vi "GET SV Variables from Target.vi"(7 "Read/Write":string, 8 "error in (no error)":errorcluster, 11 "Target":string) -> (0 "error out":errorcluster, 3 "Channel Array":refnum<class "ChannelVS.lvclass">[](array[class]))   [LabVIEW 2020, in "Shared Variables CD 2.0 Configuration.lvlib"]
uses:
  Shared Variables CD 2.0 Configuration.lvlib
  ChannelVS/ChannelVS.lvclass
  <vilib>/NI VeriStand/Custom Device API/Custom Device Item Ref.ctl
  ChannelVS/ChannelVS.lvclass/ChannelVS.ctl
  IPAddress Functions/ValidIPAddr.vi
  <vilib>/Utility/error.llb/Error Cluster From Error Code.vi
  Shared/SV Global.vi
  <resource>/objmgr/ni.var.rc
  built/windows/Channel.lvlibp/Channel.lvclass
  <vilib>/Utility/Data Type/NI_Data Type.lvlib
  <vilib>/NI VeriStand/Custom Device API/Custom Device API.lvlib
  C:/Users/Administrator/Desktop/GIT/Shared-Variable-Custom-Device-2.0/Source/built/windows/Channel.lvlibp/Channel.lvclass
panel:
  # "Loading....."
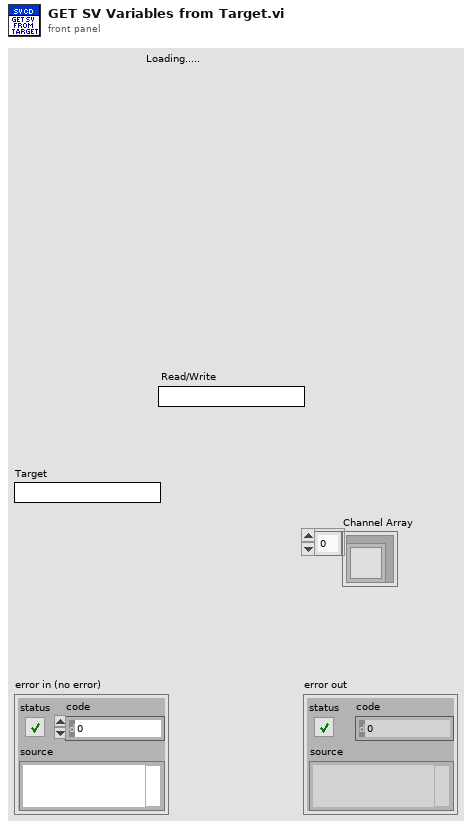
[diagram p1: front panel]
types:
  T1 = typedef "Custom Device API.lvlib/Custom Device Item Ref.ctl" = u64
  T2 = typedef "NI_Data Type.lvlib/Data Type.ctl" = enum8{"Invalid Type", "Void", "I8", "I16", "I32", "I64", "U8", "U16", "U32", "U64", "Single Float", "Double Float", "Extended Float", "Single Complex", "Double Complex", "Extended Complex", "Enum U8", "Enum U16", "Enum U32", "Enum U64", "Single Float With Unit", "Double Float With Unit", "Extended Float With Unit", "Single Complex with Unit", "Double Complex with Unit", "Extended Complex with Unit", "Boolean", "String", "Path", "Picture", "Tag", "Array", "Cluster", "Variant", "LV Variant", "Waveform", "Timestamp", "Digital Waveform", "Digital Data", "ExpressData", "Refnum", "External Data", "VI", "Poly VI", "LabVIEW Class Instance", "Fixed Point", "Set Collection", "Map Collection"}
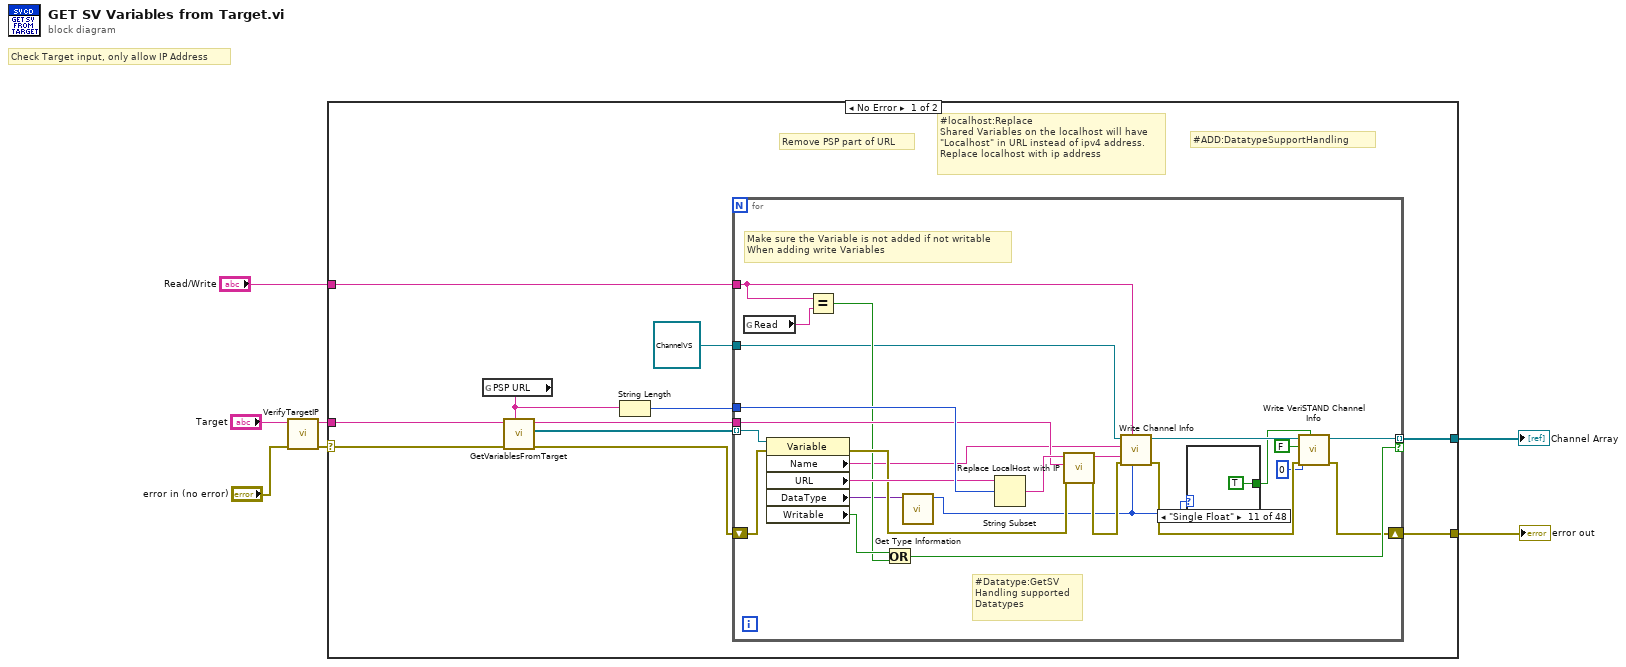
[diagram p0: block diagram]
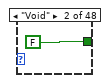
[diagram p3: hidden frame]
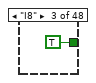
[diagram p4: hidden frame]
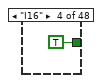
[diagram p5: hidden frame]
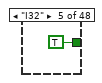
[diagram p6: hidden frame]
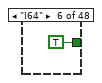
[diagram p7: hidden frame]
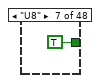
[diagram p8: hidden frame]
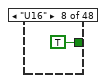
[diagram p9: hidden frame]
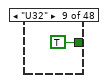
[diagram p10: hidden frame]
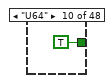
[diagram p11: hidden frame]
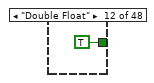
[diagram p12: hidden frame]
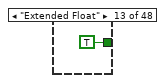
[diagram p13: hidden frame]
diagram:
  # "Check Target input, only allow IP Address"
  n1 = call "VerifyTargetIP.vi"("error in (no error)"="error in (no error)", "Target"="Target") -> ("error out"=w4:errorcluster, "IP Address String out"=w3:string)  [unwired: 8 in]
  n2 = case shown="No Error" w4 {
    selector: w4 -> [w10 w57]
    tunnel: w3 -> [w14 _]
    tunnel: [w17 w57] -> w7
    tunnel: [w16 refnum<class "ChannelVS.lvclass">[] []] -> w1
    tunnel: "Read/Write" -> [w9 _]
    frame No Error {
      # "#ADD:DatatypeSupportHandling"
      # "#localhost:Replace\nShared Variables on the localhost will have\n\"Localhost\" in URL instead of ipv4 address.\nReplace localhost with ip address"
      # "Remove PSP part of URL"
      n3 = global read "SV Global.vi" "PSP URL"() -> (w11:string)
      n4 = call "GetVariablesFromTarget.vi"("PSP URL(ni.var.psp://)"=w11, "error in (no error)"=w10, "IP Address String in"=w14) -> ("error out"=w18:errorcluster, "AllVariables[]"=w13:refnum<k21>[], "IP Address String out"=w12:string)  [unwired: 6 in]
      n5 = String Length(string=w11) -> (length=w15:i32)
      n6 = for {
        shift-right: [w22] -> w17
        shift-left: w18 -> [w43]
        tunnel: [w24] -> w16 mode=indexing if=w28
        tunnel: w15 -> [w42]
        tunnel: w13 -> [w38] mode=indexing
        tunnel: w12 -> [w37]
        tunnel: w9 -> [w30]
        tunnel: refnum<class "ChannelVS.lvclass"> refnum ("Shared Variables CD 2.0 Configuration.lvlib:ChannelVS.lvclass") -> [w29]
        # "Make sure the Variable is not added if not writable\nWhen adding write Variables"
        # "#Datatype:GetSV\nHandling supported\nDatatypes"
        n7 = global read "SV Global.vi" "Read"() -> (w35:string)
        n8 = property class="Variable"(reference=w38, error in=w43) -> (error out=w39:errorcluster, "Name"=w32:string, "URL"=w41:string, "DataType"=w27:variant, "Writable"=w36:bool)  [unwired: 1 out]
        n9 = Equal?(x=w30, y=w35) -> (x = y?=w34:bool)
        n10 = Or(x=w36, y=w34) -> (x .or. y?=w28:bool)
        n11 = call <vilib>:"Get Type Information.vi"("variant"=w27) -> ("type"=w26:T2)  [unwired: 6 in, 4 out]
        n12 = String Subset(string=w41, offset (0)=w42) -> (substring=w40:string)  [unwired: 1 in]
        n13 = call "Replace LocalHost with IP.vi"("error in (no error)"=w39, "IP Address"=w37, "URL"=w40) -> ("error out"=w31:errorcluster, "URL with IP"=w33:string)  [unwired: 7 in]
        n14 = call "Write Channel Info.vi"("DataType"=w26, "Read or Write"=w30, "error in (no error)"=w31, "URL"=w33, "Name"=w32, "Channel in"=w29) -> ("error out"=w23:errorcluster, "Channel out"=w25:refnum<class "ChannelVS.lvclass">)  [unwired: 4 in]
        n15 = case shown="\"Single Float\"" w26 {
          tunnel: [_ FALSE TRUE TRUE TRUE TRUE TRUE TRUE TRUE TRUE TRUE TRUE TRUE _ _ _ _ _ _ _ _ _ _ _ _ _ _ _ _ _ _ _ _ _ _ _ _ _ _ _ _ _ _ _ _ _ _ _] -> w21
          frame "Invalid Type", Default {
          }
          frame "Void" {
          }
          frame "I8" {
          }
          frame "I16" {
          }
          frame "I32" {
          }
          frame "I64" {
          }
          frame "U8" {
          }
          frame "U16" {
          }
          frame "U32" {
          }
          frame "U64" {
          }
          frame "Single Float" {
          }
          frame "Double Float" {
          }
          frame "Extended Float" {
          }
          frame "Single Complex" {
          }
          frame "Double Complex" {
          }
          frame "Extended Complex" {
          }
          frame "Enum U8" {
          }
          frame "Enum U16" {
          }
          frame "Enum U32" {
          }
          frame "Enum U64" {
          }
          frame "Single Float With Unit" {
          }
          frame "Double Float With Unit" {
          }
          frame "Extended Float With Unit" {
          }
          frame "Single Complex with Unit" {
          }
          frame "Double Complex with Unit" {
          }
          frame "Extended Complex with Unit" {
          }
          frame "Boolean" {
          }
          frame "String" {
          }
          frame "Path" {
          }
          frame "Picture" {
          }
          frame "Tag" {
          }
          frame "Array" {
          }
          frame "Cluster" {
          }
          frame "Variant" {
          }
          frame "LV Variant" {
          }
          frame "Waveform" {
          }
          frame "Timestamp" {
          }
          frame "Digital Waveform" {
          }
          frame "Digital Data" {
          }
          frame "ExpressData" {
          }
          frame "Refnum" {
          }
          frame "External Data" {
          }
          frame "VI" {
          }
          frame "Poly VI" {
          }
          frame "LabVIEW Class Instance" {
          }
          frame "Fixed Point" {
          }
          frame "Set Collection" {
          }
          frame "Map Collection" {
          }
        }
        n16 = call "Write VeriSTAND Channel Info.vi"("Supported in CD"=w21, "error in (no error)"=w23, "VeriSTAND Reference"=T1 0, "Exist in VeriSTAND"=FALSE, "ChannelVS in"=w25) -> ("error out"=w22:errorcluster, "ChannelVS out"=w24:refnum<class "ChannelVS.lvclass">)  [unwired: 5 in]
      }
    }
    frame Error {
    }
  }
  "error out" <- w7
  "Channel Array" <- w1
